vi "GF_status.vi"(7 "modIdTag":string="F1", 8 "error in (no error)":errorcluster, 11 "channel":refnum<k24>) -> (0 "error out":errorcluster, 1 "MotorFaultStatus":bool, 2 "CurrPosition":sgl, 3 "MotorRunState":i32(ring) items=["RunUnspecified", "RunStop", "RunForward", "RunReverse"])   [LabVIEW 2021]
uses:
  F:/2PhotonVision/psychometric_function_v2/lib/Grpc.Core.dll
  lib/Grpc.Core.dll
  F:/2PhotonVision/psychometric_function_v2/lib/FossilProtosSharp.dll
  lib/FossilProtosSharp.dll
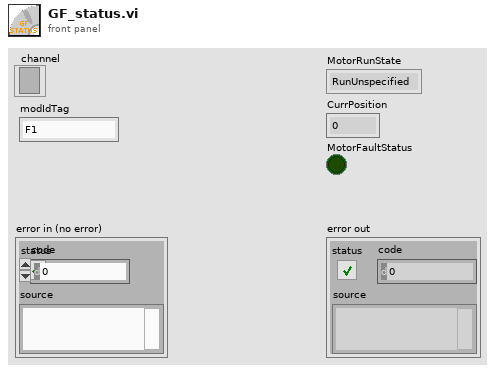
[diagram p1: front panel]
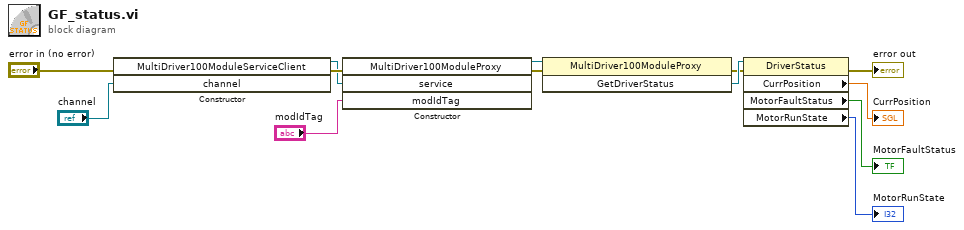
[diagram p0: block diagram]
diagram:
  n1 = constructor class="MultiDriver100ModuleServiceClie"(error in="error in (no error)", "channel"="channel") -> (reference out=w7:refnum<k24>, error out=w8:errorcluster)  [unwired: 2 in, 2 out]
  n2 = constructor class="MultiDriver100ModuleProxy"(error in=w8, "service"=w7, "modIdTag"="modIdTag") -> (reference out=w10:refnum<k24>, error out=w9:errorcluster)  [unwired: 2 in, 3 out]
  n3 = invoke class="MultiDriver100ModuleProxy" method="GetDriverStatus"(reference=w10, error in=w9) -> (error out=w5:errorcluster, "GetDriverStatus"=w6:refnum<k24>)  [unwired: 1 in, 1 out]
  n4 = property class="DriverStatus"(reference=w6, error in=w5) -> (error out=→"error out":errorcluster, "CurrPosition"=→"CurrPosition":sgl, "MotorFaultStatus"=→"MotorFaultStatus":bool, "MotorRunState"=→"MotorRunState":i32)  [unwired: 1 out]
